vi "destroy.vi"(0 "vector_weviate in":refnum<class "vector_weviate.lvclass">, 11 "error in (no error)":errorcluster) -> (4 "vector_weviate out":refnum<class "vector_weviate.lvclass">, 15 "error out":errorcluster)   [LabVIEW 2020, in "vector_weviate.lvclass"]
uses:
  vector_weviate.lvclass
  vector_weviate.lvclass/vector_weviate.ctl
  abstract_vector_base/abstract_vector_base.lvclass
  <vilib>/httpClient/LabVIEWHTTPClient.lvlib
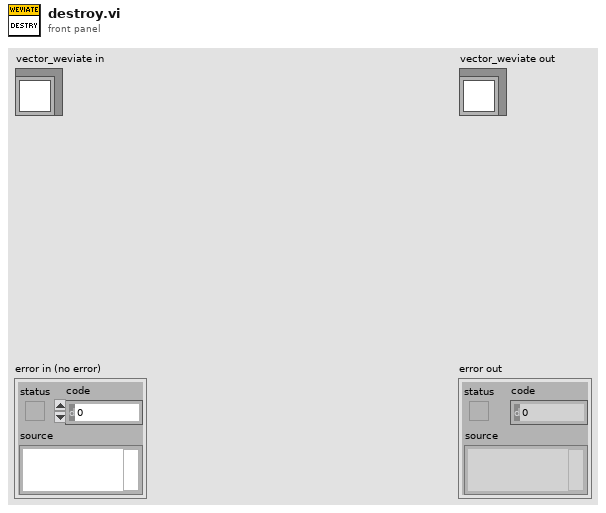
[diagram p1: front panel]
types:
  T1 = typedef "LabVIEWHTTPClient.lvlib/ClientHandle.ctl" = refnum<k1>
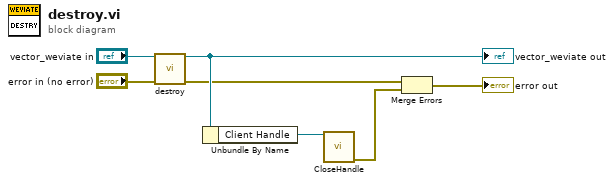
[diagram p0: block diagram]
diagram:
  n1 = call-parent "destroy.vi"("abstract_vector_base in"="vector_weviate in", "error in (no error)"="error in (no error)") -> ("abstract_vector_base out"=w5:refnum<class "vector_weviate.lvclass">, "error out"=w3:errorcluster)  [unwired: 12 in]
  "vector_weviate out" <- w5
  n2 = Unbundle By Name(w5) -> ("Client Handle"=w4:T1)
  n3 = call <vilib>:"CloseHandle.vi"("client handle"=w4) -> ("error out"=w2:errorcluster)  [unwired: 14 in]
  n4 = Merge Errors(w3, w2) -> (→"error out":errorcluster)
